vi "Get Tree Items.vi"(8 "error in (no error)":errorcluster, 10 "Filter":T1, 11 "Result Model In":refnum<class "Result Model.lvclass">) -> (0 "error out":errorcluster, 2 "Tree Items":T2(array[cluster]))   [LabVIEW 2020, in "Result Model.lvclass"]
uses:
  Result Model.lvclass
  Tree Item Filter.ctl
  Result Model.lvclass/Result Model.ctl
  Core/Result/Status.ctl
  Core/Result/Result.lvlib
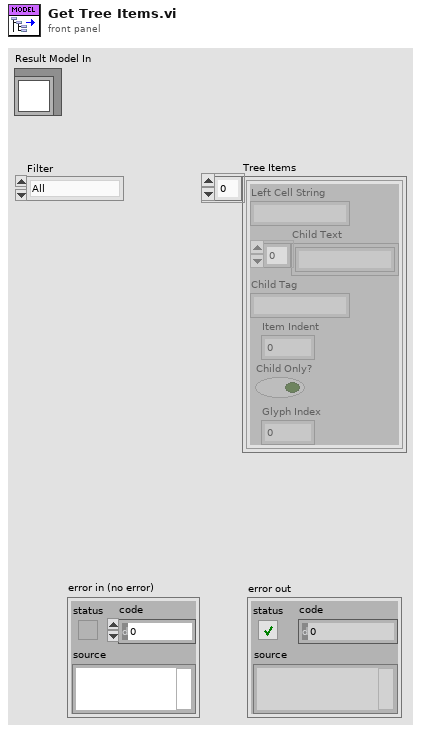
[diagram p1: front panel]
types:
  T1 = typedef "Result Model.lvclass/Tree Item Filter.ctl" = enum16{"All", "Only Fails", "Fails or else Not Executed"}
  T2 = cluster{"Left Cell String":string, "Child Text":string[], "Child Tag":string, "Item Indent":i32, "Child Only?":bool, "Glyph Index":i32}[]
  T3 = typedef "Result.lvlib/Status.ctl" = enum16{"", "Passed", "Failed", "Error", "Skipped", "Setup Error", "Broken", "Teardown Error"}
  T4 = cluster{"Left Cell String":string, "Child Text":string[], "Child Tag":string, "Item Indent":i32, "Child Only?":bool, "Glyph Index":i32}
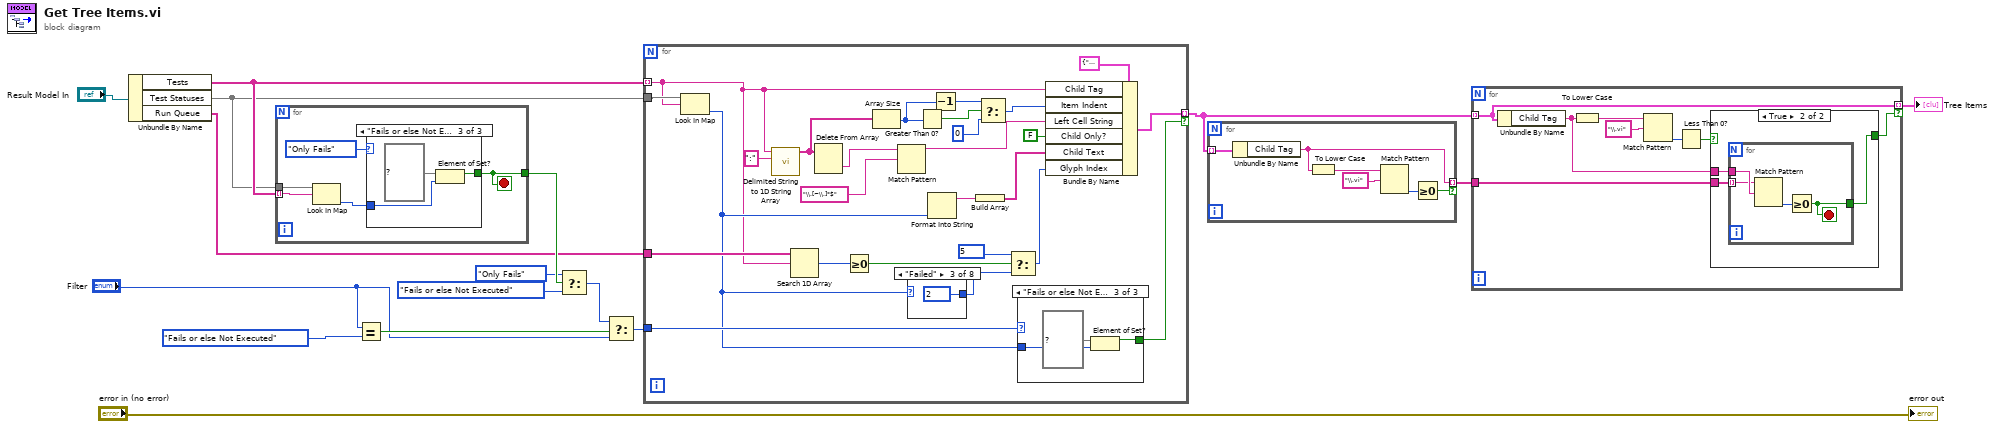
[diagram p0: block diagram]
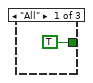
[diagram p2: hidden frame]
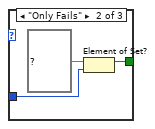
[diagram p3: hidden frame]
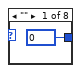
[diagram p4: hidden frame]
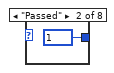
[diagram p5: hidden frame]
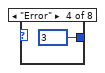
[diagram p6: hidden frame]
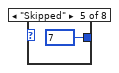
[diagram p7: hidden frame]
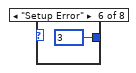
[diagram p8: hidden frame]
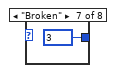
[diagram p9: hidden frame]
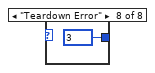
[diagram p10: hidden frame]
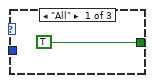
[diagram p11: hidden frame]
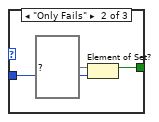
[diagram p12: hidden frame]
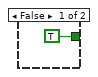
[diagram p13: hidden frame]
diagram:
  n1 = Unbundle By Name("Result Model In") -> ("Tests"=w2:string[], "Test Statuses"=w1:map{string, T3}, "Run Queue"=w3:string[])
  n2 = for {
    tunnel: [w20] -> w8
    tunnel: w2 -> [w18] mode=indexing
    tunnel: w1 -> [w19]
    stop <- w20 stop-if-true
    n3 = Look In Map(map=w19, key=w18) -> (value=w17:T3)  [unwired: 1 in, 1 out]
    n4 = case shown="\"Fails or else Not Executed\"" Tree_Item_Filter."Only Fails" ("Filter") {
      tunnel: w17 -> [_ w25 w28]
      tunnel: [TRUE w24 w27] -> w20
      frame "All" {
      }
      frame "Only Fails" {
        n5 = Element of Set?(10:w25, 11:set{T3} {enum."Failed", enum."Error", enum."Setup Error", enum."Broken", enum."Teardown Error"} ("set out")) -> (3:w24:bool)
      }
      frame "Fails or else Not Executed" {
        n6 = Element of Set?(10:w28, 11:set{T3} {enum."", enum."Failed", enum."Error", enum."Setup Error", enum."Broken", enum."Teardown Error"} ("set out")) -> (3:w27:bool)
      }
    }
  }
  n7 = Equal?(x="Filter", y=Tree_Item_Filter."Fails or else Not Executed") -> (x = y?=w10:bool)
  n8 = Select(t=Tree_Item_Filter."Only Fails" ("Filter"), s=w8, f=Tree_Item_Filter."Fails or else Not Executed" ("y")) -> (s? t:f=w5:T1)
  n9 = Select(t=w5, s=w10, f="Filter") -> (s? t:f=w12:T1)
  n10 = for {
    tunnel: [w53] -> w16 mode=indexing if=w42
    tunnel: w3 -> [w34]
    tunnel: w12 -> [w43]
    tunnel: w2 -> [w29] mode=indexing
    tunnel: w1 -> [w31]
    n11 = Look In Map(map=w31, key=w29) -> (value=w30:T3)  [unwired: 1 in, 1 out]
    n12 = call <vilib>:"Delimited String to 1D String Array.vi"("delimiter"=":", "delimited string"=w29) -> ("string array"=w49:string[])  [unwired: 9 in]
    n13 = Search 1D Array(1D array=w34, element=w29) -> (index of element=w33:i32)  [unwired: 1 in]
    n14 = Delete From Array(array=w49) -> (deleted portion=w36:string)  [unwired: 2 in, 1 out]
    n15 = Greater Or Equal To 0?(x=w33) -> (x >= 0?=w32:bool)
    n16 = Array Size(array=w49) -> (size(s)=w40:i32)
    n17 = Match Pattern(string=w36, regular expression="\\.[~\\.]*$") -> (before substring=w50:string)  [unwired: 1 in, 3 out]
    n18 = case shown="\"Failed\"" w30 {
      tunnel: [0 ("Listbox Symbol Ring Constant") 1 ("Listbox Symbol Ring Constant") 2 ("Listbox Symbol Ring Constant") 3 ("Listbox Symbol Ring Constant") 7 ("Listbox Symbol Ring Constant") 3 ("Listbox Symbol Ring Constant") 3 ("Listbox Symbol Ring Constant") 3 ("Listbox Symbol Ring Constant")] -> w44
      frame "" {
      }
      frame "Passed" {
      }
      frame "Failed" {
      }
      frame "Error" {
      }
      frame "Skipped" {
      }
      frame "Setup Error" {
      }
      frame "Broken" {
      }
      frame "Teardown Error" {
      }
    }
    n19 = Greater Than 0?(x=w40) -> (x > 0?=w41:bool)
    n20 = Format Into String(w30) -> (resulting string=w48:string)  [unwired: 3 in, 1 out]
    n21 = Decrement(x=w40) -> (x-1=w39:i32)
    n22 = Build Array(w48) -> (w47:string[])
    n23 = Select(t=w39, s=w41, f=0) -> (s? t:f=w38:i32)
    n24 = Select(t=5 ("Listbox Symbol Ring Constant"), s=w32, f=w44) -> (s? t:f=w45:i32)
    n25 = case shown="\"Fails or else Not Executed\"" w43 {
      tunnel: w30 -> [_ w66 w69]
      tunnel: [TRUE w65 w68] -> w42
      frame "All" {
      }
      frame "Only Fails" {
        n26 = Element of Set?(10:w66, 11:set{T3} {enum."Failed", enum."Error", enum."Setup Error", enum."Broken", enum."Teardown Error"} ("set out")) -> (3:w65:bool)
      }
      frame "Fails or else Not Executed" {
        n27 = Element of Set?(10:w69, 11:set{T3} {enum."", enum."Failed", enum."Error", enum."Setup Error", enum."Broken", enum."Teardown Error"} ("set out")) -> (3:w68:bool)
      }
    }
    n28 = Bundle By Name(cluster=T4 {"Left Cell String"="", "Child Text"=[], "Child Tag"="", "Item Indent"=0, "Child Only?"=FALSE, "Glyph Index"=0} ("Item"), "Child Tag"=w29, "Item Indent"=w38, "Left Cell String"=w50, "Child Only?"=FALSE, "Child Text"=w47, "Glyph Index"=w45) -> (w53:T4)
  }
  n29 = for {
    tunnel: w16 -> [w75] mode=indexing
    tunnel: [w70] -> w4 mode=indexing if=w71
    n30 = Unbundle By Name(w75) -> ("Child Tag"=w70:string)
    n31 = To Lower Case(string=w70) -> (all lower case string=w73:string)
    n32 = Match Pattern(string=w73, regular expression="\\.vi") -> (offset past match=w72:i32)  [unwired: 1 in, 3 out]
    n33 = Greater Or Equal To 0?(x=w72) -> (x >= 0?=w71:bool)
  }
  n34 = for {
    tunnel: w16 -> [w83] mode=indexing
    tunnel: [w83] -> w14 mode=indexing if=w76
    tunnel: w4 -> [w77]
    n35 = Unbundle By Name(w83) -> ("Child Tag"=w78:string)
    n36 = To Lower Case(string=w78) -> (all lower case string=w81:string)
    n37 = Match Pattern(string=w81, regular expression="\\.vi") -> (offset past match=w80:i32)  [unwired: 1 in, 3 out]
    n38 = Less Than 0?(x=w80) -> (x < 0?=w79:bool)
    n39 = case shown="True" w79 {
      tunnel: w78 -> [_ w87]
      tunnel: w77 -> [_ w86]
      tunnel: [TRUE w85] -> w76
      frame False {
      }
      frame True {
        n40 = for {
          tunnel: w87 -> [w91]
          tunnel: [w89] -> w85
          tunnel: w86 -> [w88] mode=indexing
          stop <- w89 stop-if-true
          n41 = Match Pattern(string=w88, regular expression=w91) -> (offset past match=w90:i32)  [unwired: 1 in, 3 out]
          n42 = Greater Or Equal To 0?(x=w90) -> (x >= 0?=w89:bool)
        }
      }
    }
  }
  "Tree Items" <- w14
  "error out" <- "error in (no error)"
